vi "Read Additional Labels from File.vi"(8 "error in (no error)":errorcluster, 10 "Full File Contents in":string[][](array[string]), 11 "Control Info in":refnum<class "Control Info.lvclass">) -> (0 "error out":errorcluster, 2 "Full File Contents out":string[][](array[string]), 3 "Control Info out":refnum<class "Control Info.lvclass">, 5 "Control Present in File":bool)   [LabVIEW 2017, in "Localization.lvlib" / "Control Info.lvclass"]
doc: "Reads all of the Default and Alternate Text label information from the Excel file for the specified Control when the <B>Full File Contents in</B> is empty. Otherwise the information in the <B>Full File Contents in</B> control is used. This allows for being able to read in the data once from the Excel file instead of doing it for every control or indicator.\n\nChoose Movement Consulting, LLC"
uses:
  Control Info.lvclass
  Control Info.lvclass/Control Info.ctl
  cbc32cbc-268e-45b5-b265-c4fd0a3a1155.vi
  <vilib>/addons/_office/excel.llb/Excel Get Data ([str]).vi
  <vilib>/Utility/NIReport.llb/NI_report.lvclass
  <vilib>/addons/_office/NI_ReportGenerationToolkit.lvlib
  <vilib>/Utility/NIReport.llb/Excel/NI_Excel.lvclass
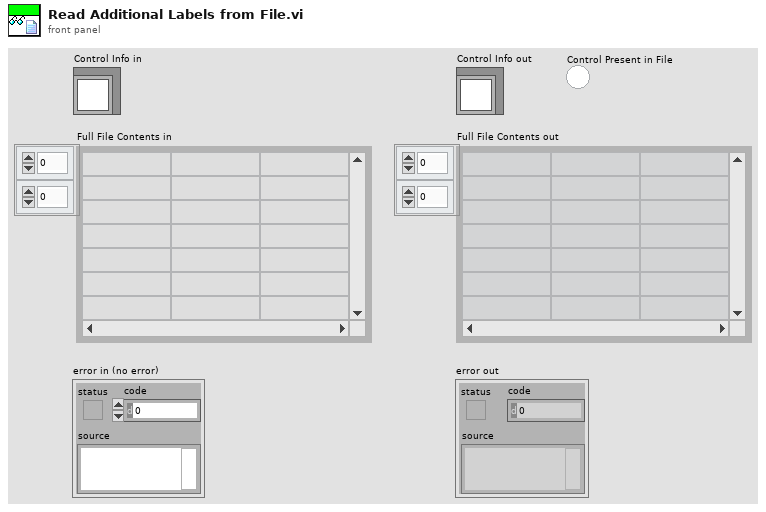
[diagram p1: front panel]
types:
  T1 = enum16{"maximized", "minimized", "normal", "no change"}
  T2 = enum16{"Standard Report", "HTML", "Word", "Excel"}
  T3 = typedef "Semaphore RefNum" = refnum<k1>
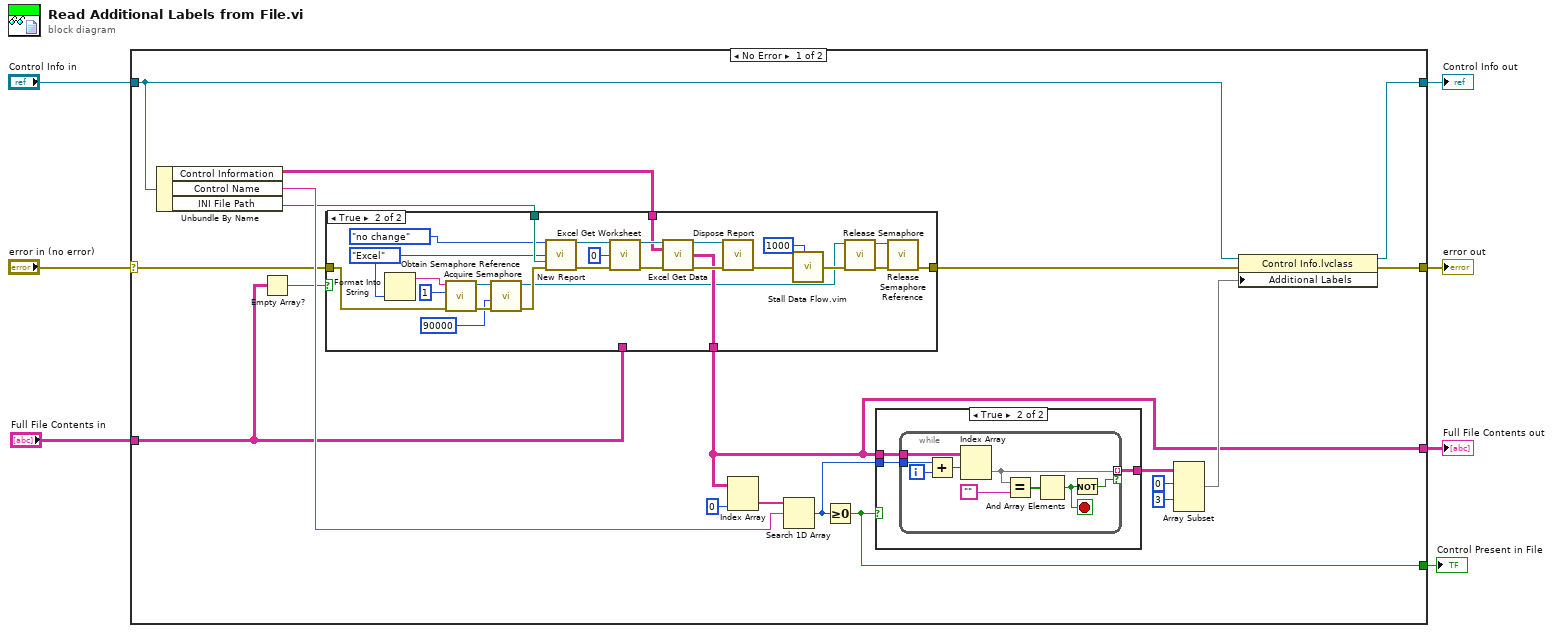
[diagram p0: block diagram]
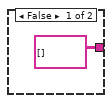
[diagram p3: hidden frame]
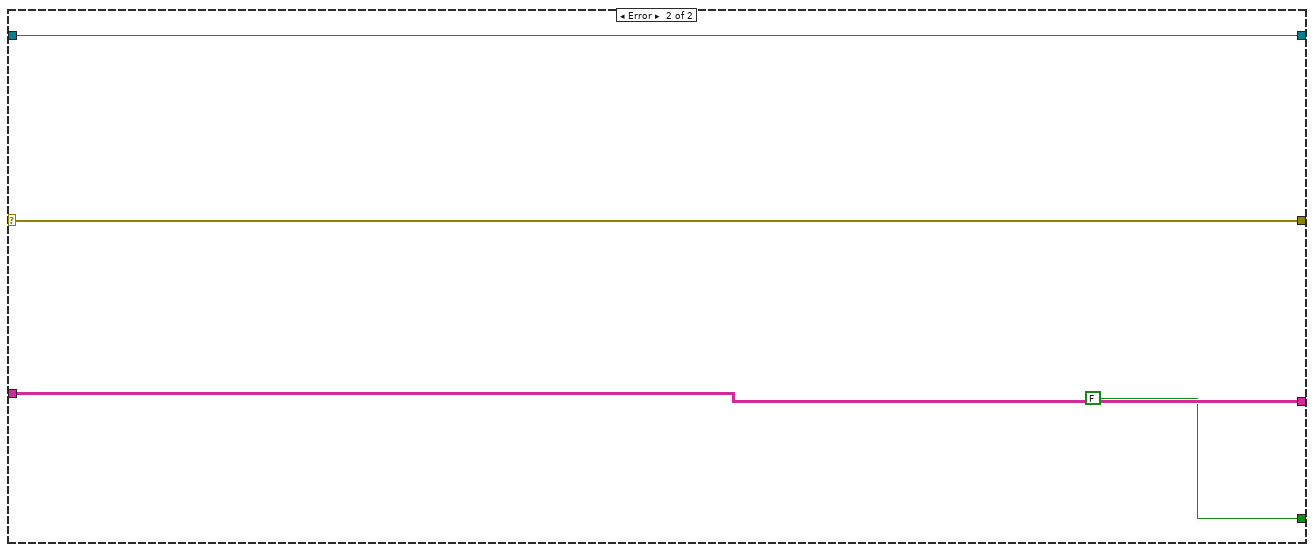
[diagram p4: hidden frame]
diagram:
  n1 = case shown="No Error" "error in (no error)" {
    selector: "error in (no error)" -> [w24 w71]
    tunnel: [w21 w71] -> w6
    tunnel: [w20 w70] -> w4
    tunnel: "Control Info in" -> [w19 w70]
    tunnel: [w17 w69] -> w3
    tunnel: "Full File Contents in" -> [w15 w69]
    tunnel: [w14 FALSE] -> w1
    frame No Error {
      n2 = Unbundle By Name(w19) -> ("Control Information"=w22:string[][], "Control Name"=w26:string, "INI File Path"=w23:path)
      n3 = Empty Array?(array=w15) -> (empty?=w16:bool)
      n4 = case shown="True" w16 {
        tunnel: w24 -> [w28 w37]
        tunnel: w23 -> [_ w54]
        tunnel: w22 -> [_ w48]
        tunnel: [w28 w30] -> w25
        tunnel: [w27 w45] -> w17
        tunnel: w15 -> [w27 _]
        frame False {
        }
        frame True {
          w29 = T2."Excel" ("report type")
          n5 = Format Into String(w29) -> (resulting string=w41:string)  [unwired: 3 in, 1 out]
          n6 = call <vilib>:"Obtain Semaphore Reference.vi"("error in (no error)"=w37, "size (1)"=1, "name (unnamed)"=w41) -> ("error out"=w43:errorcluster, "semaphore"=w42:T3)  [unwired: 2 in, 1 out]
          n7 = call <vilib>:"Acquire Semaphore.vi"("error in (no error)"=w43, "ms timeout (-1)"=90000, "semaphore"=w42) -> ("error out"=w38:errorcluster, "semaphore out"=w32:T3)  [unwired: 2 in, 1 out]
          n8 = call <vilib>:"New Report.vi"("window state (normal)"=T1."no change", "report type"=w29, "template (empty)"=w54, "error in (no error)"=w38) -> ("report out"=w53:refnum<class "NI_report.lvclass">, "error out"=w52:errorcluster)  [unwired: 10 in]
          n9 = call <vilib>:"Excel Get Worksheet.vi"("report in"=w53, "worksheet index (0)"=0, "error in (no error)"=w52) -> ("report out"=w49:refnum<class "NI_report.lvclass">, "error out"=w50:errorcluster)  [unwired: 11 in]
          n10 = call-poly <vilib>:"Excel Get Data.vi"("report in"=w49, "data type"=w48, "error in (no error)"=w50) -> ("report out"=w46:refnum<class "NI_report.lvclass">, "data"=w45:string[][], "error out"=w47:errorcluster)  [unwired: 10 in]
          n11 = call-dynamic "Dispose Report.vi"("report in"=w46, "error in (no error)"=w47) -> ("error out"=w33:errorcluster)  [unwired: 13 in]
          n12 = call "Stall Data Flow.vim"("value in"=w33, "milliseconds to wait"=u32 1000) -> ("value out"=w35:errorcluster)  [unwired: 1 out]
          n13 = call <vilib>:"Release Semaphore.vi"("error in (no error)"=w35, "semaphore"=w32) -> ("error out"=w34:errorcluster, "semaphore out"=w31:T3)  [unwired: 4 in]
          n14 = call <vilib>:"Release Semaphore Reference.vi"("error in (no error)"=w34, "semaphore"=w31) -> ("error out"=w30:errorcluster)  [unwired: 8 in, 1 out]
        }
      }
      n15 = Index Array(array=w17, index (col)=0 ("disabled index (col)")) -> (element=w12:string[])  [unwired: 1 in]
      n16 = Search 1D Array(1D array=w12, element=w26) -> (index of element=w11:i32)  [unwired: 1 in]
      n17 = Greater Or Equal To 0?(x=w11) -> (x >= 0?=w14:bool)
      n18 = case shown="True" w14 {
        tunnel: w17 -> [_ w58]
        tunnel: w11 -> [_ w57]
        tunnel: [string[][] [] ("data") w56] -> w10
        frame False {
        }
        frame True {
          n19 = while {
            tunnel: w58 -> [w67]
            tunnel: w57 -> [w66]
            tunnel: [w63] -> w56 mode=indexing if=w59
            i -> [w64]
            stop <- w60 stop-if-true
            n20 = Add(x=w66, y=w64) -> (x+y=w65:i32)
            n21 = Index Array(array=w67, index (row)=w65) -> (element=w63:string[])  [unwired: 1 in]
            n22 = Equal?(x=w63, y="") -> (x = y?=w61:bool[])
            n23 = And Array Elements(Boolean array=w61) -> (logical AND=w60:bool)
            n24 = Not(x=w60) -> (.not. x?=w59:bool)
          }
        }
      }
      n25 = Array Subset(array=w10, index (row)=0 ("index"), index (col)=3 ("index")) -> (w18:string[][])  [unwired: 2 in]
      n26 = property class="Control Info.lvclass"(reference=w19, error in=w25, "Additional Labels"=w18) -> (reference out=w20:refnum<class "Control Info.lvclass">, error out=w21:errorcluster)
    }
    frame Error {
    }
  }
  "error out" <- w6
  "Control Info out" <- w4
  "Full File Contents out" <- w3
  "Control Present in File" <- w1
